vi "Terranova908A_read_pressure.vi"(0 "VISA resource name":refnum<visa-resource-name>="COM1", 11 "error in (no error)":errorcluster) -> (4 "VISA resource name out":refnum<visa-resource-name>, 6 "pressure":dbl, 8 "pressure 2":dbl, 10 "read buffer":string, 15 "error out":errorcluster)   [LabVIEW 2015]
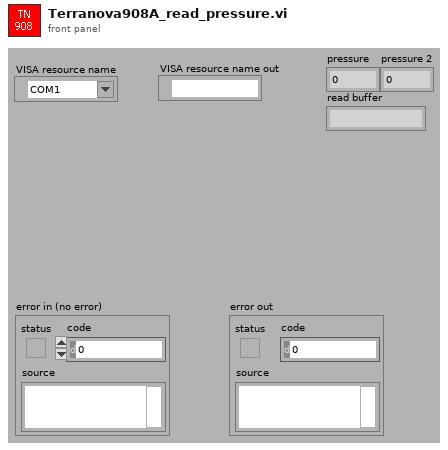
[diagram p1: front panel]
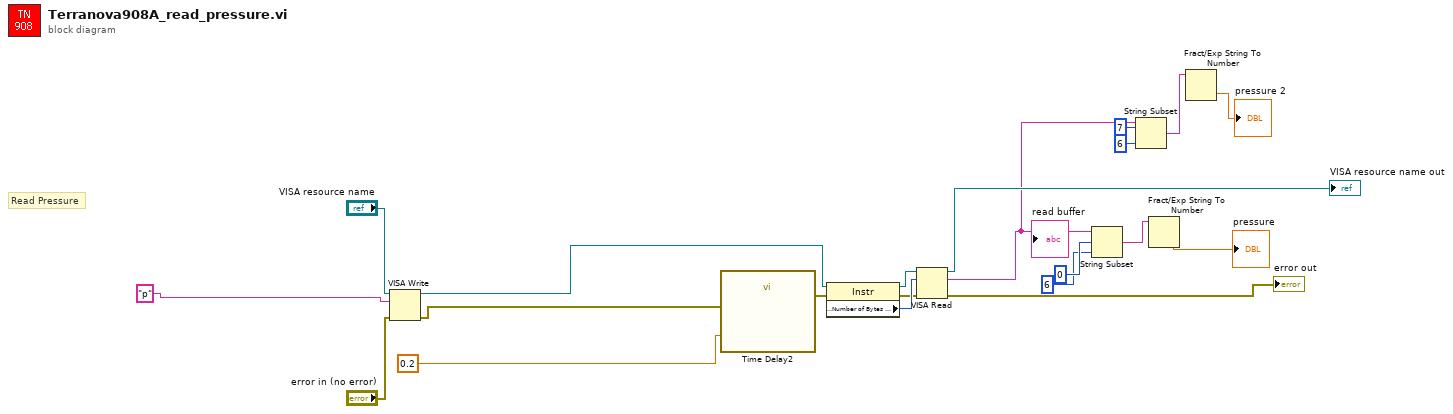
[diagram p0: block diagram]
diagram:
  # "Read Pressure"
  n1 = VISA Write(VISA resource name="VISA resource name", write buffer="p", error in (no error)="error in (no error)") -> (VISA resource name out=w14:refnum<visa-resource-name>, error out=w13:errorcluster)  [unwired: 1 out]
  n2 = call "Time Delay2"("error in (no error)"=w13, "Delay Time (s)"=0.2) -> ("error out"=w16:errorcluster)  [unwired: 9 in]
  n3 = property class="Instr"(reference=w14, error in=w16) -> (reference out=w18:refnum<visa-resource-name>, error out=w17:errorcluster, "Serial Settings:Number of Bytes at Serial Port"=w19:u32)
  n4 = VISA Read(VISA resource name=w18, byte count=w19, error in (no error)=w17) -> (VISA resource name out=→"VISA resource name out":refnum<visa-resource-name>, read buffer=w6:string, error out=→"error out":errorcluster)  [unwired: 1 out]
  "read buffer" <- w6
  n5 = String Subset(string=w6, offset (0)=0, length (rest)=6 ("length (rest)")) -> (substring=w7:string)
  n6 = String Subset(string=w6, offset (0)=7, length (rest)=6 ("length (rest)")) -> (substring=w3:string)
  n7 = Fract/Exp String To Number(string=w7) -> (number=→"pressure":dbl)  [unwired: 3 in, 1 out]
  n8 = Fract/Exp String To Number(string=w3) -> (number=→"pressure 2":dbl)  [unwired: 3 in, 1 out]
